vi "WVFM_to_File.vi"(7 "LVWSR":refnum<class "Web Request.lvclass">, 11 "Write_Data":u8) -> ()   [LabVIEW 2014]
uses:
  <vilib>/wsapi/Web Request.lvclass
  Controller/Messages/Stop PAS Wvfm Write MSG/Stop PAS Wvfm Write MSG.lvclass
  Controller/Messages/Start PAS Wvfm File MSG/Start PAS Waveform File MSG.lvclass
  Controller/Controller.lvclass
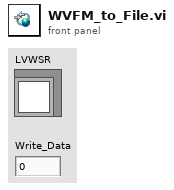
[diagram p1: front panel]
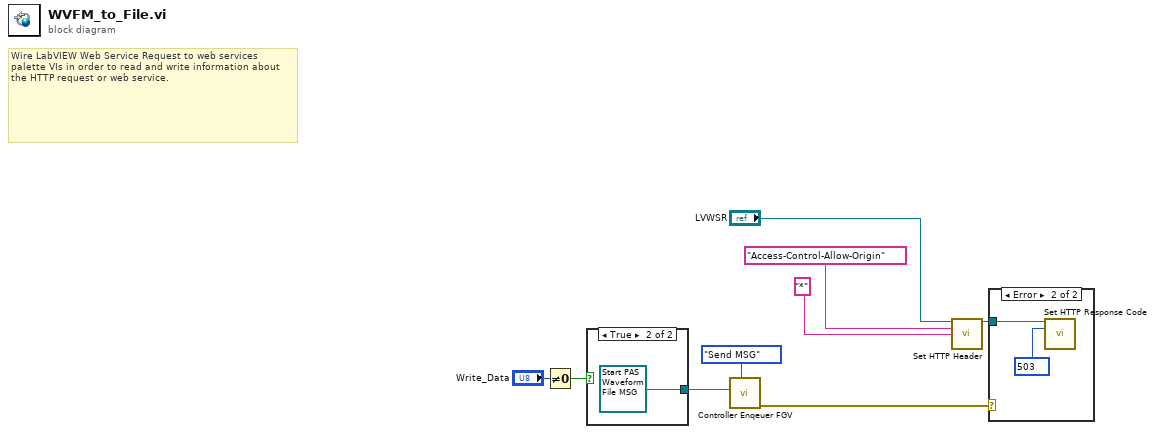
[diagram p0: block diagram]
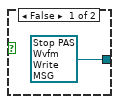
[diagram p2: hidden frame]
diagram:
  # "Wire LabVIEW Web Service Request to web services palette VIs in order to read and write information about the HTTP request or web service."
  n1 = Not Equal To 0?(x="Write_Data") -> (x != 0?=w4:bool)
  n2 = case shown="True" w4 {
    tunnel: [refnum<class "Stop PAS Wvfm Write MSG.lvclass"> refnum ("Controller:Stop PAS Wvfm Write MSG.lvclass") refnum<class "Start PAS Waveform File MSG.lvclass"> refnum ("Controller:Start Calibration")] -> w3
    frame False {
    }
    frame True {
    }
  }
  n3 = call "Controller Enqeuer FGV.vi"("State"=enum16{"Store", "Send MSG"}."Send MSG", "MSG"=w3) -> ("error out"=w2:errorcluster)  [unwired: 9 in]
  n4 = call <vilib>:"Set HTTP Header.vi"("LabVIEW Web Service Request"="LVWSR", "header"="Access-Control-Allow-Origin", "header value"="*") -> ("LabVIEW Web Service Request out"=w6:refnum<class "Web Request.lvclass">)  [unwired: 11 in, 1 out]
  n5 = case shown="Error" w2 {
    tunnel: w6 -> [_ w13]
    frame No Error {
    }
    frame Error {
      w12 = 503 items=["100"=100, "101"=101, "200"=200, "201"=201, "202"=202, "203"=203, "204"=204, "205"=205, "206"=206, "300"=300, "301"=301, "302"=302, "303"=303, "304"=304, "305"=305, "306"=306, "307"=307, "400"=400, "401"=401, "402"=402, "403"=403, "404"=404, "405"=405, "406"=406, "407"=407, "408"=408, "409"=409, "410"=410, "411"=411, "412"=412, "413"=413, "414"=414, "415"=415, "416"=416, "417"=417, "500"=500, "501"=501, "502"=502, "503"=503, "504"=504, "505"=505] ("response code (200)")
      n6 = call <vilib>:"Set HTTP Response Code.vi"("LabVIEW Web Service Request"=w13, "response code (200)"=w12) -> ()  [unwired: 12 in, 2 out]
    }
  }
